vi "LWXPS_RequestType2.vi"(0 "XPS Reference IN":refnum<k24>, 11 "LabVIEW error IN":errorcluster) -> (3 "XPS Reference OUT":refnum<k24>, 4 "Returned error code":i32, 6 "Header":string, 8 "Time Stamp":string, 10 "Zygo Laser Power":string, 14 "LabVIEW error OUT":errorcluster, 15 "XPS Error String":string)   [LabVIEW 2014]
uses:
  D:/XPSQ8_LabView_Library/Development/Source/Dll/Newport.XPS.CommandInterface.dll
  Dll/Newport.XPS.CommandInterface.dll
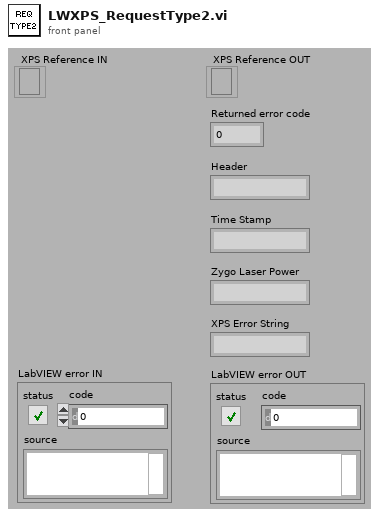
[diagram p1: front panel]
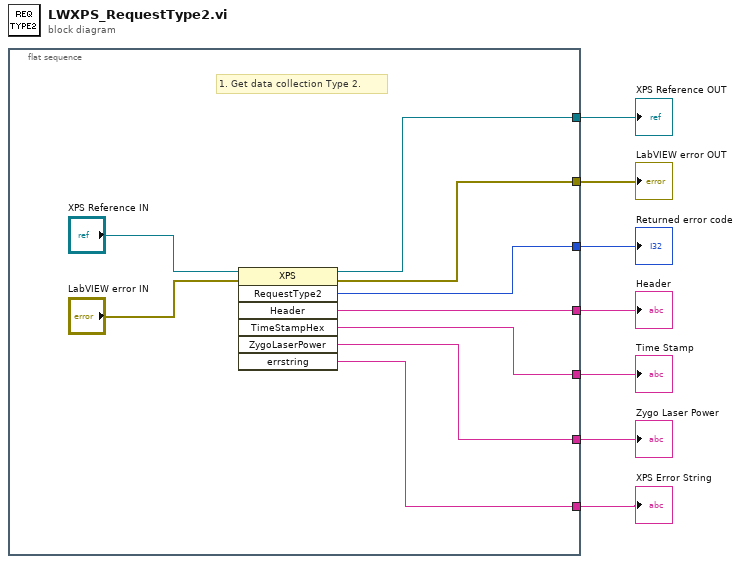
[diagram p0: block diagram]
diagram:
  n1 = flat-sequence {
    tunnel: [w15] -> w7
    tunnel: [w13] -> w6
    tunnel: [w8] -> w5
    tunnel: [w12] -> w4
    tunnel: [w11] -> w1
    tunnel: [w10] -> w3
    tunnel: [w9] -> w2
    frame #0 {
      # "1. Get data collection Type 2."
      n2 = invoke class="XPS" method="RequestType2"(reference="XPS Reference IN", error in="LabVIEW error IN") -> (reference out=w15:refnum<k24>, error out=w13:errorcluster, "RequestType2"=w8:i32, "Header"=w9:string, "TimeStampHex"=w12:string, "ZygoLaserPower"=w11:string, "errstring"=w10:string)  [unwired: 5 in]
    }
  }
  "XPS Error String" <- w3
  "XPS Reference OUT" <- w7
  "LabVIEW error OUT" <- w6
  "Returned error code" <- w5
  "Time Stamp" <- w4
  "Header" <- w2
  "Zygo Laser Power" <- w1
